vi "Test CTL class.vi"() -> ()   [LabVIEW 2012]
uses:
  ctl_class/ctl.lvclass
  <vilib>/LAVA/UI Tools/Fading/_Fade(I32)__lava_lib_ui_tools.vi
panel:
  in  "Templates":i32(listbox)
  in  "500ms toggle":bool=TRUE
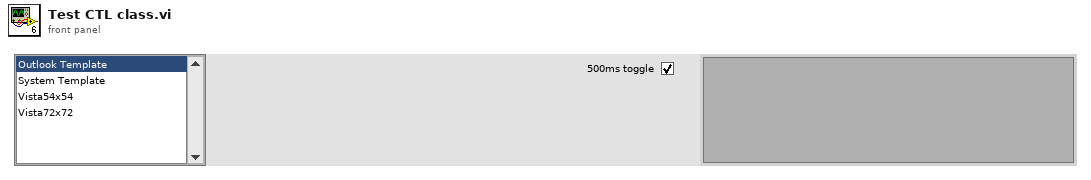
[diagram p1: front panel]
types:
  T1 = enum32{"invalid app kind", "Development System", "Run Time System", "Student Edition", "Embedded LabVIEW", "Evaluation", "Custom"}
  T2 = enum32{"Invalid", "Standard", "Closed", "Hidden", "Minimized", "Maximized"}
  T3 = cluster{"Core":cluster{"Current VI Reference":refnum<vi>, "Close Panel on Exit?":bool}, "MenuLaunch":cluster{"App":refnum<vi>, "VI Name":string, "menu launched?":bool}}
  T4 = cluster{"App":refnum<vi>, "VI Name":string, "menu launched?":bool}
  T5 = cluster{"Current VI Reference":refnum<vi>, "Close Panel on Exit?":bool}
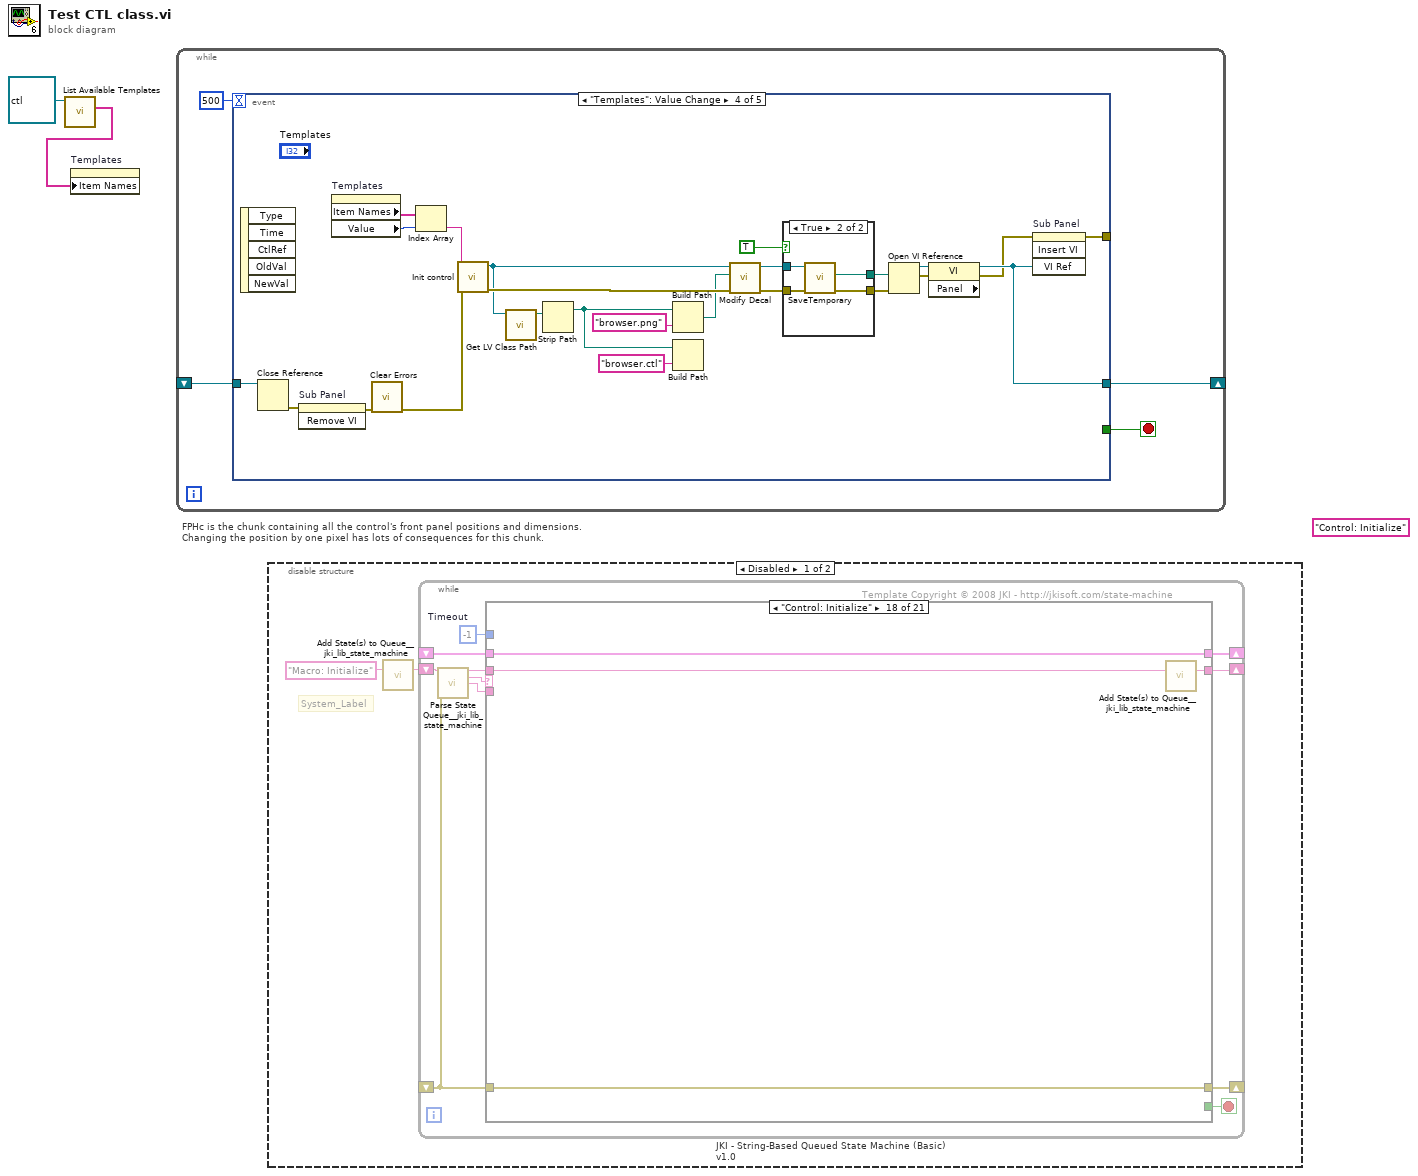
[diagram p0: block diagram]
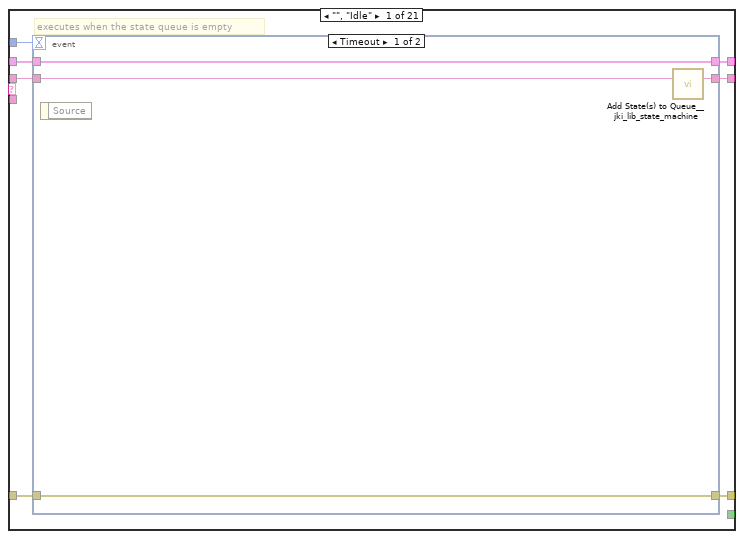
[diagram p2: hidden frame]
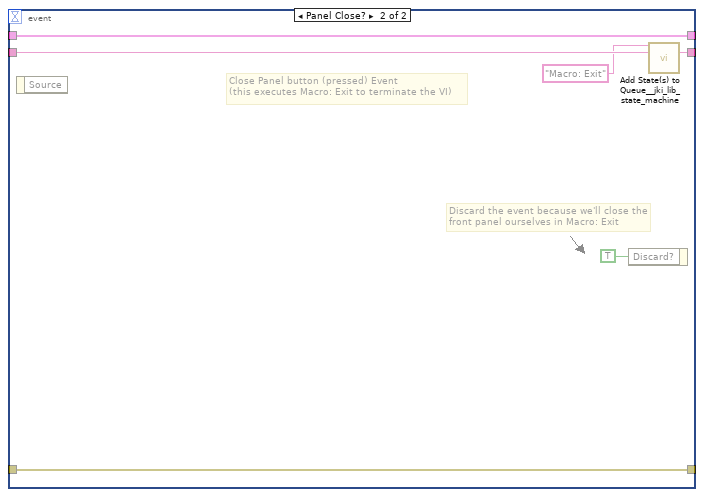
[diagram p3: hidden frame]
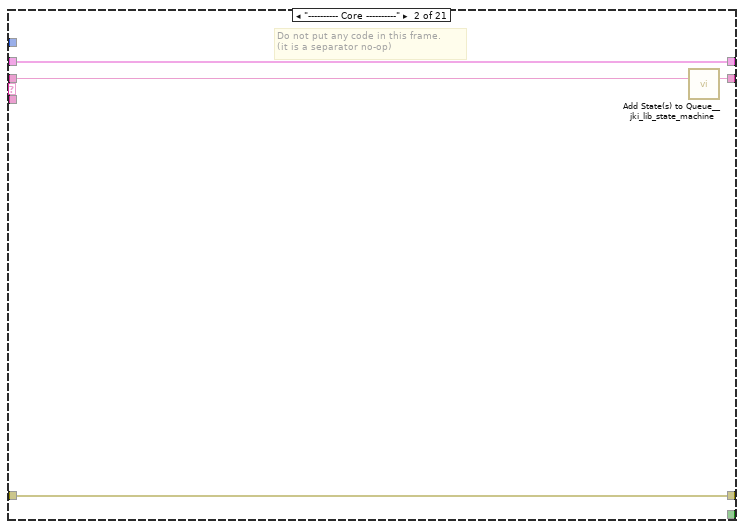
[diagram p4: hidden frame]
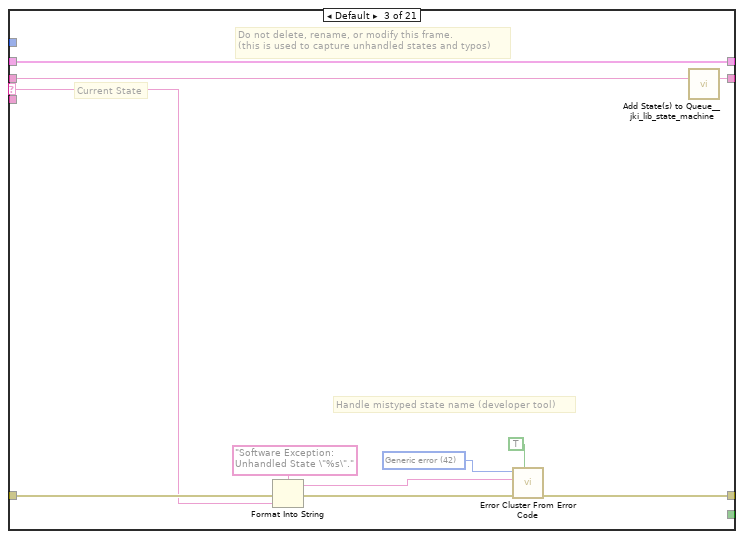
[diagram p5: hidden frame]
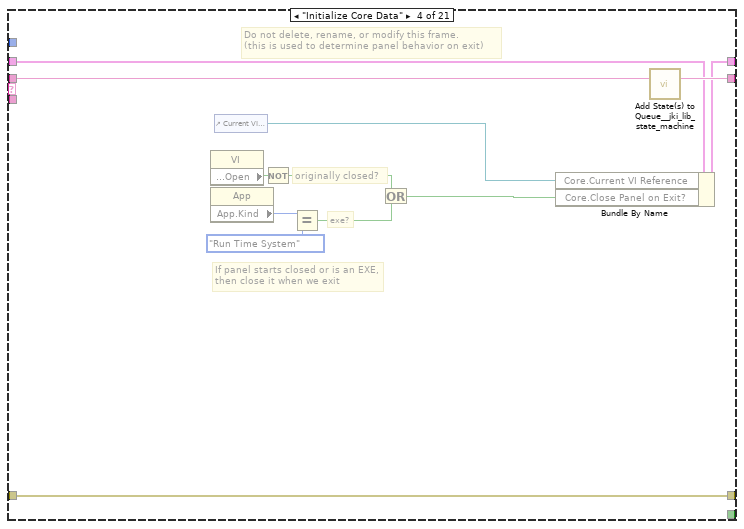
[diagram p6: hidden frame]
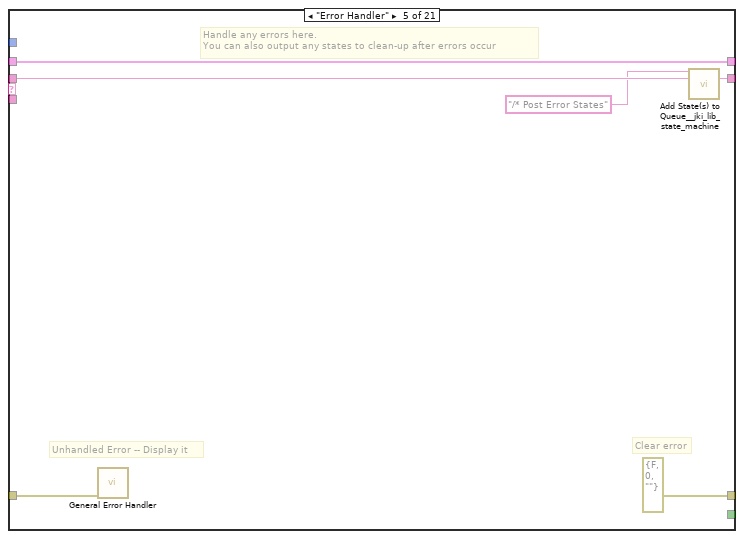
[diagram p7: hidden frame]
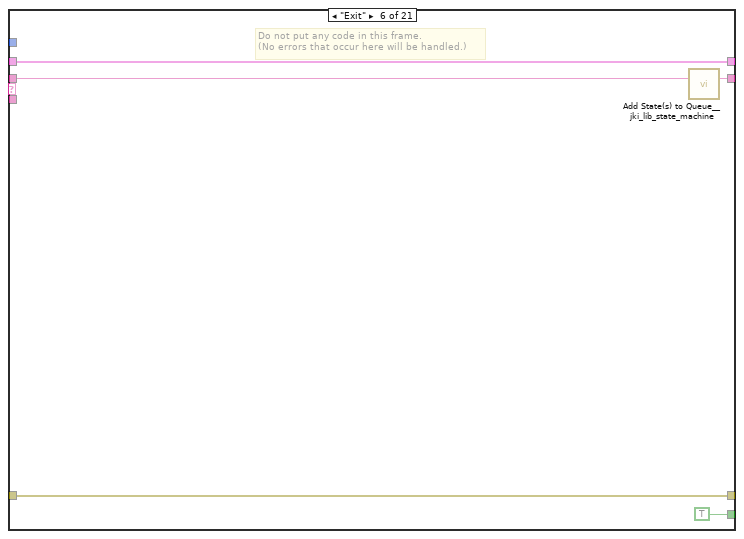
[diagram p8: hidden frame]
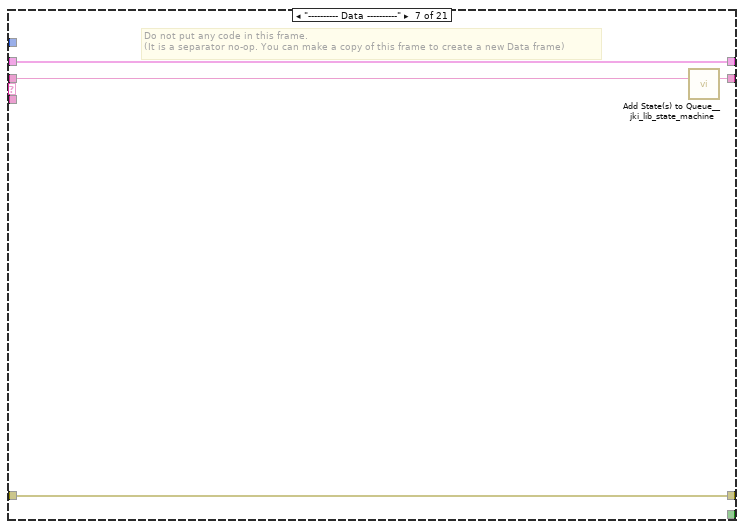
[diagram p9: hidden frame]
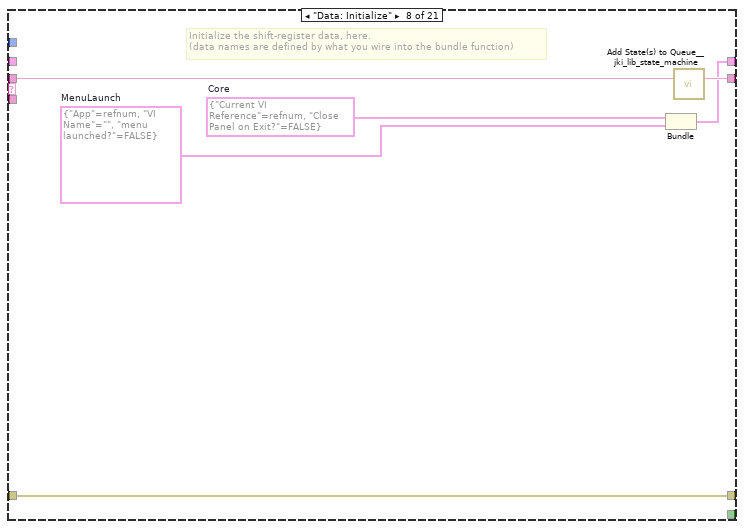
[diagram p10: hidden frame]
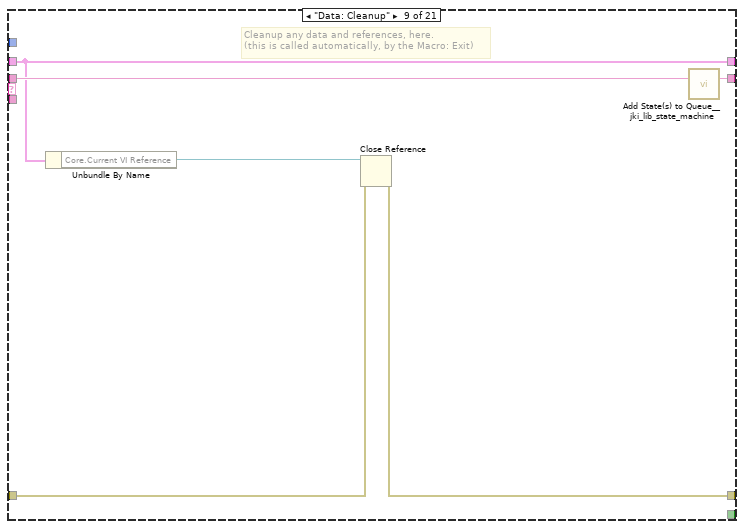
[diagram p11: hidden frame]
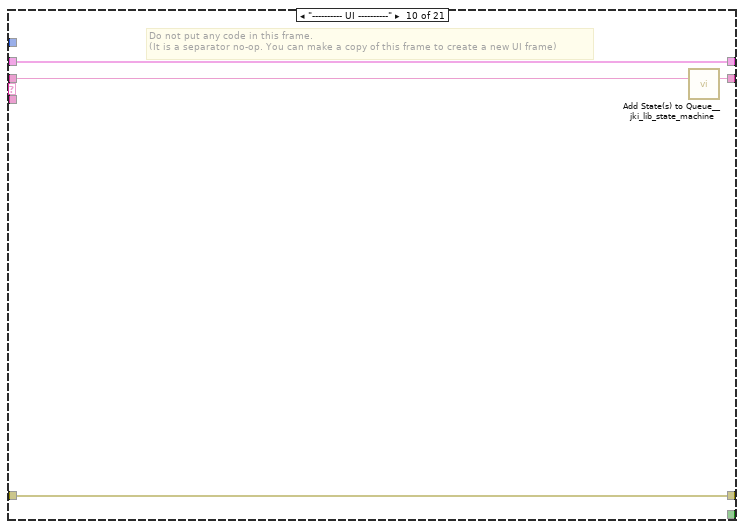
[diagram p12: hidden frame]
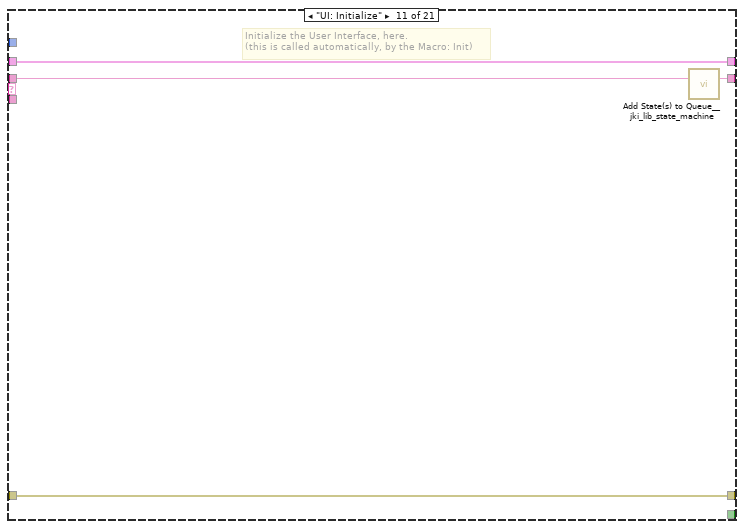
[diagram p13: hidden frame]
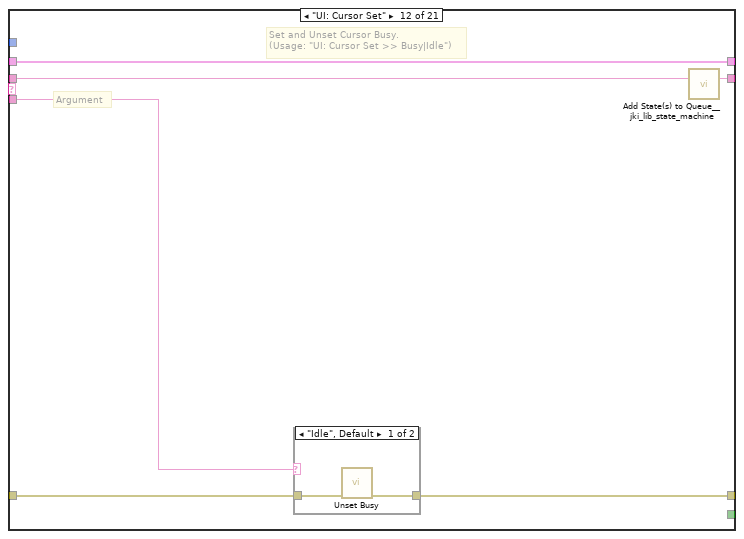
[diagram p14: hidden frame]
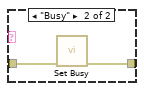
[diagram p15: hidden frame]
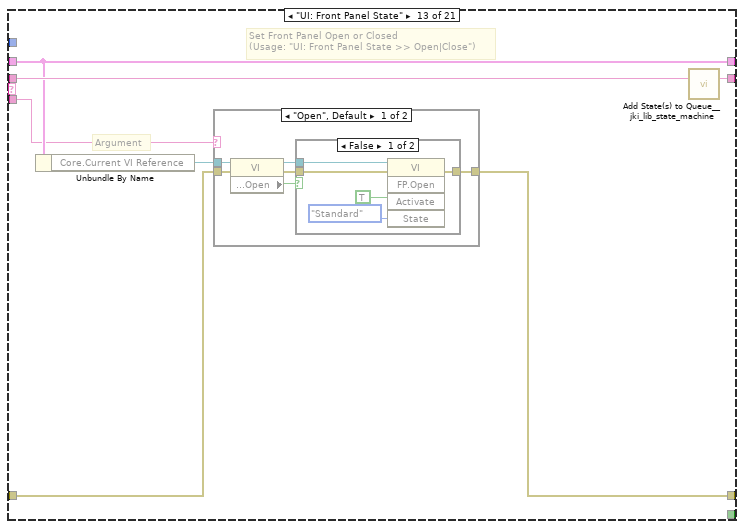
[diagram p16: hidden frame]
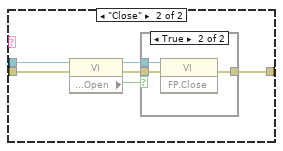
[diagram p18: hidden frame]
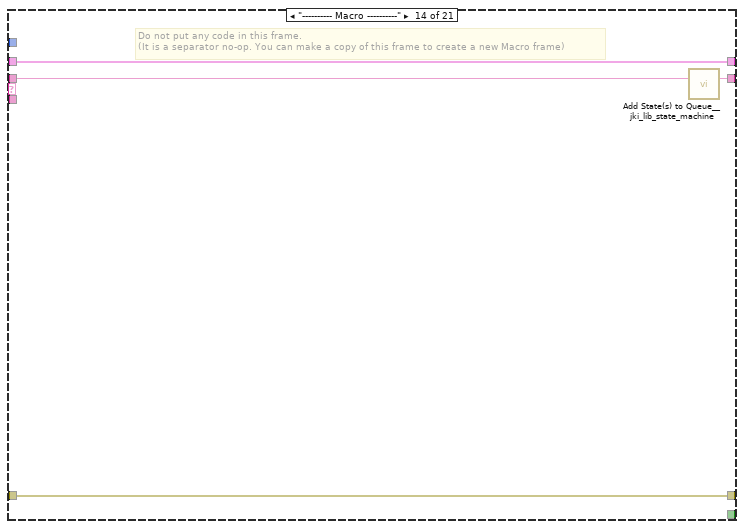
[diagram p20: hidden frame]
diagram:
  (unwired) "Control: Initialize"
  # "FPHc is the chunk containing all the control's front panel positions and dimensions.\nChanging the position by one pixel has lots of consequences for this chunk."
  n1 = call "List Available Templates.vi"("ctl in"=refnum<class "ctl.lvclass"> refnum) -> ("Templates Available"=w1:string[])  [unwired: 7 in, 3 out]
  n2 = property on="Templates" class="LstBox (strict)"("Item Names"=w1) -> ()  [unwired: 2 in, 2 out]
  n3 = while {
    shift-right: [w3] -> _
    shift-left: _ -> [w4]
    stop <- w5 stop-if-true
    n4 = event shown="[3] \"Templates\": Value Change" {
      selector: _ -> [_ _ _ _ _]
      dyn-events: _ -> [_ _ _ _ _]
      timeout: 500 -> [_ _ _ _ _]
      tunnel: [_ _ w35 _ _] -> w5
      tunnel: w4 -> [w8 w30 w34 w46 w65]
      tunnel: [w7 w30 w34 w44 w65] -> w3
      tunnel: [_ _ _ w39 _] -> _
      event Timeout {
        n5 = event-data() -> ()  [unwired: 1 in, 2 out]
        n6 = case shown="True" "500ms toggle" {
          tunnel: w8 -> [w10 w21]
          tunnel: [w10 w19] -> w7
          frame False {
          }
          frame True {
            n7 = property class="VI"(reference=w21) -> (reference out=w19:refnum<vi>, error out=w12:errorcluster, "Panel"=w20:refnum<vi>)  [unwired: 1 in]
            n8 = property class="Pnl"(reference=w20, error in=w12) -> (error out=w11:errorcluster, "Controls[]"=w18:refnum<vi>[])  [unwired: 1 out]
            n9 = Index Array(array=w18) -> (element=w17:refnum<vi>)  [unwired: 1 in]
            n10 = feedback #1(TRUE) -> (w15:bool)
            n11 = Not(x=w15) -> (.not. x?=w14:bool)
            n12 = feedback-in #1(w14) -> ()
            n13 = property class="Ctl"(reference=w17, error in=w11, "Value"=w14) -> (error out=w13:errorcluster)  [unwired: 1 out]
            n14 = call <vilib>:"Clear Errors.vi"("error in (no error)"=w13) -> ()  [unwired: 6 in, 1 out]
          }
        }
      }
      event VI Activation {
        n15 = event-data() -> ("VIName"=w27:string, "AppRef"=w22:refnum<vi>, "VIAppRef"=w26:refnum<vi>)  [unwired: 1 in]
        n16 = control-ref of="This VI"() -> (w29:refnum<vi>)
        n17 = property class="VI"(reference=w29) -> ("Name"=w28:string)  [unwired: 1 in, 2 out]
        n18 = Equal?(x=w28, y=w27) -> (x = y?=w24:bool)
        n19 = Equal?(x=w22, y=w26) -> (x = y?=w25:bool)
        n20 = And(x=w24, y=w25) -> (x .and. y?=w23:bool)
        n21 = case shown="True" w23 {
          frame False {
            n22 = call-poly <vilib>:"Fade (Polymorphic)__lava_lib_ui_tools.vi"("Target Transparency (0)"=u8 25, "Fade time (ms)"=250) -> ()  [unwired: 8 in, 2 out]
          }
          frame True {
            n23 = call-poly <vilib>:"Fade (Polymorphic)__lava_lib_ui_tools.vi"("Fade time (ms)"=250) -> ()  [unwired: 9 in, 2 out]
          }
        }
      }
      event Panel Close? {
        w35 = TRUE ("Discard?")
        n24 = event-data() -> ()  [unwired: 1 in, 3 out]
        n25 = event-data("Discard?"=w35) -> ()  [unwired: 1 in, 1 out]
      }
      event "Templates": Value Change {
        n26 = event-data() -> ()  [unwired: 1 in, 5 out]
        n27 = Close Reference(reference=w46) -> (error out=w45:errorcluster)  [unwired: 1 in]
        n28 = invoke on="Sub Panel" class="SubPanel" method="Remove VI"(error in=w45) -> (error out=w47:errorcluster)  [unwired: 2 in, 2 out]
        n29 = property on="Templates" class="LstBox (strict)"() -> ("Item Names"=w38:string[], "Value"=w37:i32)  [unwired: 2 in, 2 out]
        n30 = call <vilib>:"Clear Errors.vi"("error in (no error)"=w47) -> ("error out"=w40:errorcluster)  [unwired: 6 in]
        n31 = Index Array(array=w38, index=w37) -> (element=w36:string)
        n32 = call "Init control.vi"("error in"=w40, "Template Name"=w36) -> ("error out"=w59:errorcluster, "ctl out"=w53:refnum<class "ctl.lvclass">)  [unwired: 1 in, 7 out]
        n33 = call <vilib>:"Get LV Class Path.vi"("object"=w53) -> ("class path"=w55:path)  [unwired: 1 in, 9 out]
        n34 = Strip Path(path=w55) -> (stripped path=w51:path)  [unwired: 1 out]
        n35 = Build Path(base path=w51, name or relative path="browser.png") -> (appended path=w50:path)
        n36 = Build Path(base path=w51, name or relative path="browser.ctl") -> ()  [unwired: 1 out]
        n37 = call-dynamic "Modify Decal.vi"("error in (no error)"=w59, "new decal"=w50, "ctl in"=w53) -> ("error out"=w56:errorcluster, "ctl out"=w57:refnum<class "ctl.lvclass">)  [unwired: 7 out]
        n38 = case shown="True" TRUE {
          tunnel: w57 -> [_ w64]
          tunnel: w56 -> [w60 w63]
          tunnel: [_ w61] -> w49
          tunnel: [w60 w62] -> w48
          frame False {
          }
          frame True {
            n39 = call-dynamic "SaveTemporary.vi"("error in (no error)"=w63, "ctl in"=w64) -> ("error out"=w62:errorcluster, "Temporary Control"=w61:path)  [unwired: 7 in, 1 out]
          }
        }
        n40 = Open VI Reference(vi path=w49, error in (no error)=w48) -> (vi reference=w41:refnum<vi>, error out=w43:errorcluster)  [unwired: 4 in]
        n41 = property class="VI" props=["Panel"](reference=w41, error in=w43) -> (reference out=w44:refnum<vi>, error out=w42:errorcluster)  [unwired: 1 out]
        n42 = invoke on="Sub Panel" class="SubPanel" method="Insert VI"(error in=w42, "VI Ref"=w44) -> (error out=w39:errorcluster)  [unwired: 2 in, 3 out]
      }
      event Mouse Down {
        # "Prepare Drag of control to drop on another FP or move the decal"
        n43 = event-data() -> ()  [unwired: 1 in, 7 out]
      }
    }
  }
  n44 = disable-structure shown="Disabled" {
    frame Disabled {
      # "System_Label"
      n45 = call <vilib>:"Add State(s) to Queue__jki_lib_state_machine.vi"("State(s) in (\"\")"="Macro: Initialize") -> ("States Out"=w67:string)  [unwired: 14 in]
      n46 = while "JKI - String-Based Queued State Machine (Basic) v1.0" {
        shift-right: [w71] -> _
        shift-left: _ -> [w70]
        shift-right: [w74] -> _
        shift-left: _ -> [w68]
        shift-right: [w73] -> _
        shift-left: w67 -> [w75]
        stop <- w72 stop-if-true
        w69 = -1  # Timeout
        # "Template Copyright © 2008 JKI - http://jkisoft.com/state-machine"
        n47 = call <vilib>:"Parse State Queue__jki_lib_state_machine.vi"("State Queue"=w75, "Error In (no error)"=w68) -> ("Remaining States"=w77:string, "Current State"=w78:string, "Arguments"=w76:string)  [unwired: 11 in]
        n48 = case shown="\"Control: Initialize\"" w78 {
          selector: w78 -> [_ _ w100 _ _ _ _ _ _ _ _ _ _ _ _ _ _ _ _ _ _]
          tunnel: w77 -> [w85 w99 w104 w122 w128 w133 w137 w143 w149 w153 w157 w163 w174 w200 w205 w215 w219 w223 w227 w237 w241]
          tunnel: w76 -> [_ _ _ _ _ _ _ _ _ _ _ w158 w168 _ _ _ _ _ _ _ _]
          tunnel: w70 -> [w83 w96 w102 w113 w125 w131 w134 _ w144 w150 w155 w161 w170 w197 w202 w212 w216 w220 w224 w234 w238]
          tunnel: [w82 w97 w106 w119 errorcluster {"status"=FALSE, "code"=0, "source"=""} ("error out") w130 w135 w140 w145 w151 w154 w159 w171 w198 w203 w213 w217 w221 w225 w235 w239] -> w74
          tunnel: w68 -> [w81 w97 w105 w119 w124 w130 w135 w140 w146 w151 w154 w160 w172 w198 w203 w213 w217 w221 w225 w235 w239]
          tunnel: [w84 w98 w103 w121 w127 w132 w136 w142 w148 w152 w156 w162 w173 w199 w204 w214 w218 w222 w226 w236 w240] -> w73
          tunnel: [_ _ _ _ _ TRUE _ _ _ _ _ _ _ _ _ _ _ _ _ _ _] -> w72
          tunnel: [w80 w96 w102 w120 w125 w131 w134 w141 w144 w150 w155 w161 w170 w197 w202 w212 w216 w220 w224 w233 w238] -> w71
          tunnel: w69 -> [w79 _ _ _ _ _ _ _ _ _ _ _ _ _ _ _ _ _ _ _ _]
          frame "", "Idle" {
            # "executes when the state queue is empty"
            n49 = event shown="[0] Timeout" {
              selector: _ -> [_ _]
              dyn-events: _ -> [_ _]
              timeout: w79 -> [_ _]
              tunnel: w85 -> [w89 w95]
              tunnel: [w88 w94] -> w84
              tunnel: w83 -> [w86 w92]
              tunnel: [w87 w93] -> w82
              tunnel: w81 -> [w87 w93]
              tunnel: [w86 w92] -> w80
              event Timeout {
                n50 = event-data() -> ()  [unwired: 1 in, 1 out]
                n51 = call <vilib>:"Add State(s) to Queue__jki_lib_state_machine.vi"("State(s) in (\"\")"=w89) -> ("States Out"=w88:string)  [unwired: 14 in]
              }
              event Panel Close? {
                # "Discard the event because we'll close the front panel ourselves in Macro: Exit"
                # "Close Panel button (pressed) Event\n(this executes Macro: Exit to terminate the VI)"
                n52 = event-data() -> ()  [unwired: 1 in, 1 out]
                n53 = event-data("Discard?"=TRUE) -> ()  [unwired: 1 in, 1 out]
                n54 = call <vilib>:"Add State(s) to Queue__jki_lib_state_machine.vi"("State(s) in Front (\"\")"="Macro: Exit", "State(s) in (\"\")"=w95) -> ("States Out"=w94:string)  [unwired: 13 in]
              }
            }
          }
          frame "---------- Core ----------" {
            # "Do not put any code in this frame.\n(it is a separator no-op)"
            n55 = call <vilib>:"Add State(s) to Queue__jki_lib_state_machine.vi"("State(s) in (\"\")"=w99) -> ("States Out"=w98:string)  [unwired: 14 in]
          }
          frame Default {
            w109 = 42 items=["No error", "Argument error", "Memory is full", "Out of zone", "End of file", "File already open", "Generic file I/O error", "File not found", "File permission error", "Disk is full", "Duplicate path", "Too many files open", "System feature not enabled", "Resource file not found", "Cannot add resource", "Resource not found", "Image not found", "Image memory error", "Pen does not exist", "Config type invalid", "Config token not found", "Config parse error", "Config memory error", "Bad external code format", "Bad external code offset", "External code not present", "Null window", "Destroy window error", "Null menu", "Print aborted", "Bad print record", "Print driver error", "Windows error during printing", "Memory error during printing", "Print dialog error", "Generic print error", "Invalid device refnum", "Device not found", "Device parameter error", "Device unit error", "Cannot open device", "Device call aborted", "Generic error", "Cancelled by user", "Object ID too low", "Object ID too high", "Object not in heap", "Unknown heap", "Unknown object (invalid DefProc)", "Unknown object (DefProc not in table)", "Message out of range", "Invalid (null) method", "Unknown message", "Manager call not supported", "Bad address", "Network operation in progress", "Network operation timed out", "Connection is busy", "Network attribute not supported", "Network error", "Address in use", "System out of memory", "Connection aborted", "Connection refused", "Not connected", "Already connected", "Connection closed", "Initialization error (interapplication manager)", "Bad occurrence", "Wait on unbound occurrence handler", "Occurrence queue overflow", "Datalog type conflict", "Unused", "Unrecognized type (interapplication manager)", "Memory corrupt", "Failed to make temporary DLL", "Old CIN version", "Drag socket not found", "Failed to load drop-object", "Failed to register OLE object", "Failed to release OLE object", "Format specifier type mismatch", "Unknown format specifier", "Too few format specifiers", "Too many format specifiers", "Scan failed", "Newer CIN version", "Error converting to variant", "Runtime menu error", "Password tampered", "Variant attribute not found", "Incompatible variant data type", "Event data is not available", "Event Store is not present", "Occurrence is not found", "Event Queue is not created", "Event info is not available", "Refnum passed is NULL", "Error retrieving Class GUID", "Error retrieving CoClass GUID", "Error retrieving TypeLib GUID.", "Bad built application magic bytes.", "Specific driver is different from the specific driver associated with the Logical Name.", "There is no session opened to the class driver.", "Max Error", "MAX - Error with config objects", "MAX - Error loading configuration", "MAX - Group not supported"]
            # "Current State"
            # "Do not delete, rename, or modify this frame.\n(this is used to capture unhandled states and typos)"
            # "Handle mistyped state name (developer tool)"
            n56 = Format Into String(format string="Software Exception: Unhandled State \"%s\"." ("message"), error in=w105, w100) -> (resulting string=w108:string, error out=w107:errorcluster)  [unwired: 1 in]
            n57 = call <vilib>:"Error Cluster From Error Code.vi"("show call chain? (False)"=TRUE, "error in (no error)"=w107, "error message (\"\")"=w108, "error code (0)"=w109) -> ("error out"=w106:errorcluster)  [unwired: 5 in]
            n58 = call <vilib>:"Add State(s) to Queue__jki_lib_state_machine.vi"("State(s) in (\"\")"=w104) -> ("States Out"=w103:string)  [unwired: 14 in]
          }
          frame "Initialize Core Data" {
            # "Do not delete, rename, or modify this frame.\n(this is used to determine panel behavior on exit)"
            # "originally closed?"
            # "exe?"
            # "If panel starts closed or is an EXE, then close it when we exit"
            n59 = property class="VI"() -> ("Front Panel.Open"=w118:bool)  [unwired: 2 in, 2 out]
            n60 = property class="App"() -> ("App.Kind"=w117:T1)  [unwired: 2 in, 2 out]
            n61 = control-ref of="Current VI Reference"() -> (w111:refnum<vi>)
            n62 = Not(x=w118) -> (.not. x?=w115:bool)
            n63 = Equal?(x=w117, y=T1."Run Time System" ("Application:Kind")) -> (x = y?=w114:bool)
            n64 = Or(x=w115, y=w114) -> (x .or. y?=w112:bool)
            n65 = Bundle By Name(cluster=w113, "Core.Current VI Reference"=w111, "Core.Close Panel on Exit?"=w112) -> (w120:T3)
            n66 = call <vilib>:"Add State(s) to Queue__jki_lib_state_machine.vi"("State(s) in (\"\")"=w122) -> ("States Out"=w121:string)  [unwired: 14 in]
          }
          frame "Error Handler" {
            # "Unhandled Error -- Display it"
            # "Handle any errors here.\nYou can also output any states to clean-up after errors occur"
            # "Clear error"
            n67 = call <vilib>:"General Error Handler.vi"("error in (no error)"=w124) -> ()  [unwired: 10 in, 5 out]
            n68 = call <vilib>:"Add State(s) to Queue__jki_lib_state_machine.vi"("State(s) in Front (\"\")"="/* Post Error States", "State(s) in (\"\")"=w128) -> ("States Out"=w127:string)  [unwired: 13 in]
          }
          frame "Exit" {
            # "Do not put any code in this frame.\n(No errors that occur here will be handled.)"
            n69 = call <vilib>:"Add State(s) to Queue__jki_lib_state_machine.vi"("State(s) in (\"\")"=w133) -> ("States Out"=w132:string)  [unwired: 14 in]
          }
          frame "---------- Data ----------" {
            # "Do not put any code in this frame.\n(It is a separator no-op. You can make a copy of this frame to create a new Data frame)"
            n70 = call <vilib>:"Add State(s) to Queue__jki_lib_state_machine.vi"("State(s) in (\"\")"=w137) -> ("States Out"=w136:string)  [unwired: 14 in]
          }
          frame "Data: Initialize" {
            w138 = T4 {"App"=refnum, "VI Name"="", "menu launched?"=FALSE}  # MenuLaunch
            w139 = T5 {"Current VI Reference"=refnum, "Close Panel on Exit?"=FALSE}  # Core
            # "Initialize the shift-register data, here.\n(data names are defined by what you wire into the bundle function)"
            n71 = Bundle("Core"=w139, "MenuLaunch"=w138) -> (w141:T3)  [unwired: 1 in]
            n72 = call <vilib>:"Add State(s) to Queue__jki_lib_state_machine.vi"("State(s) in (\"\")"=w143) -> ("States Out"=w142:string)  [unwired: 14 in]
          }
          frame "Data: Cleanup" {
            # "Cleanup any data and references, here.\n(this is called automatically, by the Macro: Exit)"
            n73 = Unbundle By Name(w144) -> ("Core.Current VI Reference"=w147:refnum<vi>)
            n74 = Close Reference(reference=w147, error in (no error)=w146) -> (error out=w145:errorcluster)
            n75 = call <vilib>:"Add State(s) to Queue__jki_lib_state_machine.vi"("State(s) in (\"\")"=w149) -> ("States Out"=w148:string)  [unwired: 14 in]
          }
          frame "---------- UI ----------" {
            # "Do not put any code in this frame.\n(It is a separator no-op. You can make a copy of this frame to create a new UI frame)"
            n76 = call <vilib>:"Add State(s) to Queue__jki_lib_state_machine.vi"("State(s) in (\"\")"=w153) -> ("States Out"=w152:string)  [unwired: 14 in]
          }
          frame "UI: Initialize" {
            # "Initialize the User Interface, here.\n(this is called automatically, by the Macro: Init)"
            n77 = call <vilib>:"Add State(s) to Queue__jki_lib_state_machine.vi"("State(s) in (\"\")"=w157) -> ("States Out"=w156:string)  [unwired: 14 in]
          }
          frame "UI: Cursor Set" {
            # "Argument"
            # "Set and Unset Cursor Busy.\n(Usage: \"UI: Cursor Set >> Busy|Idle\")"
            n78 = case shown="\"Idle\", Default" w158 {
              tunnel: w160 -> [w165 w167]
              tunnel: [w164 w166] -> w159
              frame "Idle", Default {
                n79 = call <vilib>:"Unset Busy.vi"("error in (no error)"=w165) -> ("error out"=w164:errorcluster)  [unwired: 10 in]
              }
              frame "Busy" {
                n80 = call <vilib>:"Set Busy.vi"("error in (no error)"=w167) -> ("error out"=w166:errorcluster)  [unwired: 9 in, 1 out]
              }
            }
            n81 = call <vilib>:"Add State(s) to Queue__jki_lib_state_machine.vi"("State(s) in (\"\")"=w163) -> ("States Out"=w162:string)  [unwired: 14 in]
          }
          frame "UI: Front Panel State" {
            # "Argument"
            # "Set Front Panel Open or Closed\n(Usage: \"UI: Front Panel State >> Open|Close\")"
            n82 = Unbundle By Name(w170) -> ("Core.Current VI Reference"=w169:refnum<vi>)
            n83 = case shown="\"Open\", Default" w168 {
              tunnel: w172 -> [w178 w191]
              tunnel: [w180 w192] -> w171
              tunnel: w169 -> [w179 w189]
              frame "Open", Default {
                n84 = property class="VI"(reference=w179, error in=w178) -> (reference out=w176:refnum<vi>, error out=w177:errorcluster, "Front Panel.Open"=w175:bool)
                n85 = case shown="False" w175 {
                  tunnel: [w183 w186] -> w180
                  tunnel: w177 -> [w182 w186]
                  tunnel: w176 -> [w181 _]
                  frame False {
                    n86 = invoke class="VI" method="FP.Open"(reference=w181, error in=w182, "Activate"=TRUE, "State"=T2."Standard") -> (error out=w183:errorcluster)  [unwired: 1 in, 4 out]
                  }
                  frame True {
                  }
                }
              }
              frame "Close" {
                n87 = property class="VI"(reference=w189, error in=w191) -> (reference out=w188:refnum<vi>, error out=w190:errorcluster, "Front Panel.Open"=w187:bool)
                n88 = case shown="True" w187 {
                  tunnel: [w193 w196] -> w192
                  tunnel: w190 -> [w193 w195]
                  tunnel: w188 -> [_ w194]
                  frame False {
                  }
                  frame True {
                    n89 = invoke class="VI" method="FP.Close"(reference=w194, error in=w195) -> (error out=w196:errorcluster)  [unwired: 1 in, 2 out]
                  }
                }
              }
            }
            n90 = call <vilib>:"Add State(s) to Queue__jki_lib_state_machine.vi"("State(s) in (\"\")"=w174) -> ("States Out"=w173:string)  [unwired: 14 in]
          }
          frame "---------- Macro ----------" {
            # "Do not put any code in this frame.\n(It is a separator no-op. You can make a copy of this frame to create a new Macro frame)"
            n91 = call <vilib>:"Add State(s) to Queue__jki_lib_state_machine.vi"("State(s) in (\"\")"=w200) -> ("States Out"=w199:string)  [unwired: 14 in]
          }
          frame "Macro: Initialize" {
            w201 = "Data: Initialize\nInitialize Core Data\nUI: Initialize\nUI: Front Panel State >> Open\nApp.MenuLaunch"  # Data: Initialize Initialize Core Data UI: Initialize UI: Front Panel State >> Open App.MenuLaunch
            # "Initialization Macro\n(This is called once, when the VI starts)"
            n92 = call <vilib>:"Add State(s) to Queue__jki_lib_state_machine.vi"("State(s) in Front (\"\")"=w201, "State(s) in (\"\")"=w205) -> ("States Out"=w204:string)  [unwired: 13 in]
          }
          frame "Macro: Exit" {
            # "Exit Macro\n(This is called once, when the VI exits)"
            n93 = Unbundle By Name(w212) -> ("Core.Close Panel on Exit?"=w211:bool)
            n94 = Select(t="UI: Front Panel State >> Close", s=w211, f="") -> (s? t:f=w208:string)
            n95 = call <vilib>:"Add State(s) to Queue__jki_lib_state_machine.vi"("State(s) in (\"\")"=w208, "State(s) at Back (\"\")"="Data: Cleanup\nExit") -> ("States Out"=w206:string)  [unwired: 13 in]
            n96 = call <vilib>:"Add State(s) to Queue__jki_lib_state_machine.vi"("State(s) in Front (\"\")"=w206, "State(s) in (\"\")"=w215) -> ("States Out"=w214:string)  [unwired: 13 in]
          }
          frame "---------- Control ----------" {
            n97 = call <vilib>:"Add State(s) to Queue__jki_lib_state_machine.vi"("State(s) in (\"\")"=w219) -> ("States Out"=w218:string)  [unwired: 14 in]
          }
          frame "Control: Initialize" {
            n98 = call <vilib>:"Add State(s) to Queue__jki_lib_state_machine.vi"("State(s) in (\"\")"=w223) -> ("States Out"=w222:string)  [unwired: 14 in]
          }
          frame "---------- Application ----------" {
            n99 = call <vilib>:"Add State(s) to Queue__jki_lib_state_machine.vi"("State(s) in (\"\")"=w227) -> ("States Out"=w226:string)  [unwired: 14 in]
          }
          frame "App.MenuLaunch" {
            # "Your code here.\n(You can make a copy of, or modify, this frame)"
            n100 = property class="App"() -> (error out=w230:errorcluster, "App.MenuLaunchApp"=w232:refnum<vi>, "App.MenuLaunchVI"=w231:string)  [unwired: 2 in, 1 out]
            n101 = Unbundle By Name(w230) -> ("status"=w229:bool)
            n102 = Not(x=w229) -> (.not. x?=w228:bool)
            n103 = Bundle By Name(cluster=w234, "MenuLaunch.menu launched?"=w228, "MenuLaunch.App"=w232, "MenuLaunch.VI Name"=w231) -> (w233:T3)
            n104 = call <vilib>:"Add State(s) to Queue__jki_lib_state_machine.vi"("State(s) in (\"\")"=w237) -> ("States Out"=w236:string)  [unwired: 14 in]
          }
          frame "New Category: 2" {
            # "Your code here.\n(You can make a copy of, or modify, this frame)"
            n105 = call <vilib>:"Add State(s) to Queue__jki_lib_state_machine.vi"("State(s) in (\"\")"=w241) -> ("States Out"=w240:string)  [unwired: 14 in]
          }
        }
      }
    }
    frame Enabled {
    }
  }
